vi "Register.vi"(8 "error in (no error)":errorcluster, 11 "Test Executive View in":refnum<class "Test Executive View.lvclass">) -> (0 "error out":errorcluster, 3 "Test Executive View out":refnum<class "Test Executive View.lvclass">)   [LabVIEW 2017, in "Test Executive View.lvclass"]
uses:
  Test Executive View.lvclass
  <vilib>/gpm_packages/@cs/mva-core/Source/IObserver/IObserver/IObserver.lvclass
  <vilib>/gpm_packages/@cs/mva-core/Source/SubscriptionPolicy/BasicSubscription/BasicSubscription.lvclass
  Source/Test Executive Builder View/Test Executive Builder View Messages/Draw Tree Msg/Draw Tree Msg.lvclass
  C:/Users/jonmc/Documents/Git/Test Executive Builder/gpm_packages/@cs/mva-core/Source/IMediator/ISubscriptionPolicy/ISubscriptionPolicy.lvclass
  C:/Users/jonmc/Documents/Git/Test Executive Builder/gpm_packages/@cs/transport/Source/Concrete/ActorMessageTransport/Notification Msg/Notification Msg.lvclass
  C:/Users/jonmc/Documents/Git/Test Executive Builder/gpm_packages/@cs/mva-core/Source/IObserver/IObserver/IObserver.lvclass
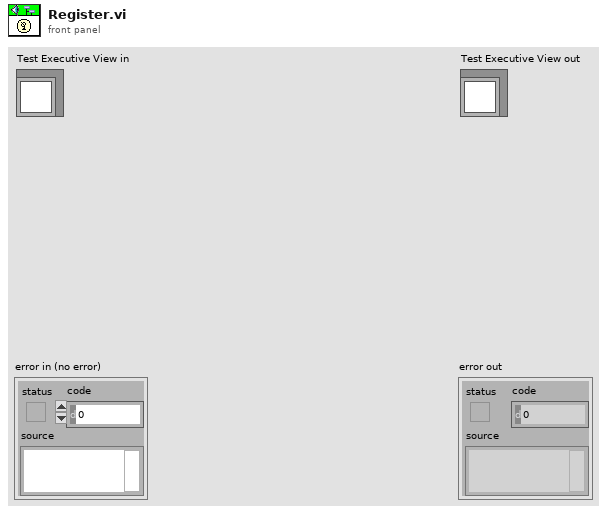
[diagram p1: front panel]
types:
  T1 = cluster{"Left Cell String":string, "Child Text":string[], "Child Tag":string, "Item Indent":i32, "Child Only?":bool, "Glyph Index":i32}[]
  T2 = typedef "IMediator.lvlib/ISubscriptionPolicy.lvclass/ISubscriptionPolicy Reference.ctl" = refnum<data-value>
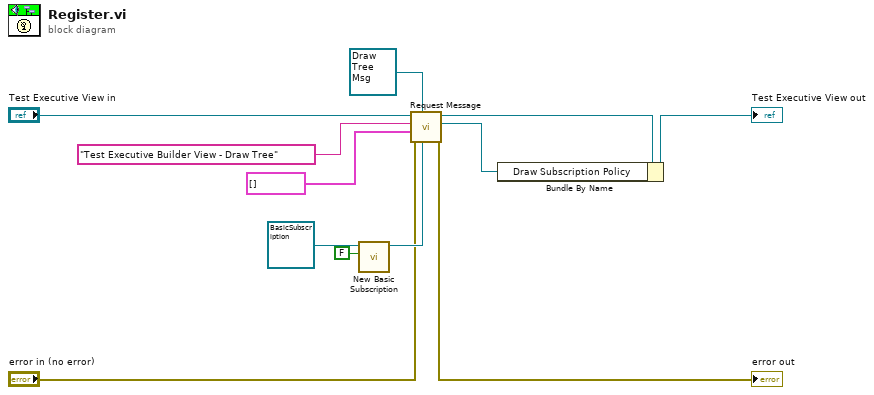
[diagram p0: block diagram]
diagram:
  n1 = call <vilib>:"New Basic Subscription.vi"("Ignore Past Updates? (F)"=FALSE, "BasicSubscription In"=refnum<class "BasicSubscription.lvclass"> refnum ("SubscriptionPolicy.lvlib:BasicSubscription.lvclass")) -> ("BasicSubscription Out"=w10:refnum<class "BasicSubscription.lvclass">)  [unwired: 9 in]
  n2 = call <vilib>:"Request Message.vi"("Configured SubscriptionPolicy"=w10, "Desired Notification Msg"=refnum<class "Draw Tree Msg.lvclass"> refnum ("Test Executive Builder View.lvlib:Draw Tree Msg.lvclass"), "error in (no error)"="error in (no error)", "Data Type"=T1 [] ("Tree Data"), "Datum Name"="Test Executive Builder View - Draw Tree", "IObserver in"="Test Executive View in") -> ("error out"=→"error out":errorcluster, "Subscription Policy"=w3:T2, "IObserver out"=w5:refnum<class "Test Executive View.lvclass">)  [unwired: 3 in]
  n3 = Bundle By Name(cluster=w5, "Draw Subscription Policy"=w3) -> (→"Test Executive View out":refnum<class "Test Executive View.lvclass">)
